vi "detAttributeString.vi"(8 "error in (no error)":errorcluster, 10 "XML In":string, 11 "ReadAttribute In":refnum<class "XMLAttributeParser.lvclass">) -> (0 "error out":errorcluster, 1 "AttributesOK?":bool, 2 "AttributeString":string, 3 "ReadAttribute Out":refnum<class "XMLAttributeParser.lvclass">)   [LabVIEW 2016, in "XML.lvlib" / "XMLAttributeParser.lvclass"]
doc: "This method determines the full attribute string to parse, and performs a quality check."
uses:
  <userlib>/Common/XML/XMLAttributeParser/XMLAttributeParser.lvclass
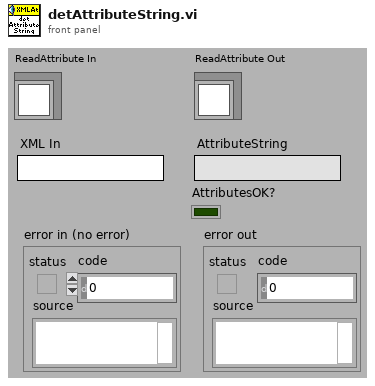
[diagram p1: front panel]
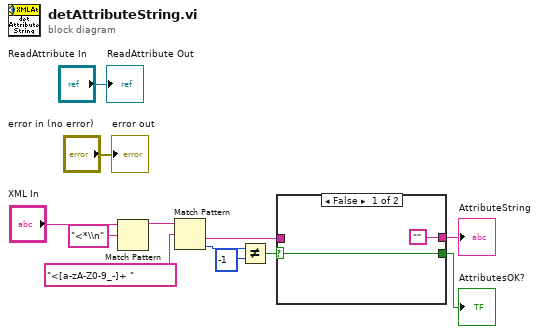
[diagram p0: block diagram]
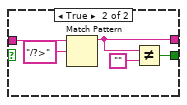
[diagram p2: hidden frame]
diagram:
  n1 = Match Pattern(string="XML In", regular expression="<*\\n") -> (before substring=w12:string)  [unwired: 1 in, 3 out]
  n2 = Match Pattern(string=w12, regular expression="<[a-zA-Z0-9_-]+ ") -> (after substring=w8:string, offset past match=w10:i32)  [unwired: 1 in, 2 out]
  n3 = Not Equal?(x=w10, y=-1) -> (x != y?=w9:bool)
  n4 = case shown="False" w9 {
    selector: w9 -> [w13 _]
    tunnel: w8 -> [_ w17]
    tunnel: [w13 w15] -> w4
    tunnel: ["" w16] -> w3
    frame False {
    }
    frame True {
      n5 = Match Pattern(string=w17, regular expression="/?>") -> (before substring=w16:string)  [unwired: 1 in, 3 out]
      n6 = Not Equal?(x=w16, y="") -> (x != y?=w15:bool)
    }
  }
  "AttributesOK?" <- w4
  "AttributeString" <- w3
  "ReadAttribute Out" <- "ReadAttribute In"
  "error out" <- "error in (no error)"
